vi "TableReceiverGoToSkill.vi"(7 "Firstcall?":bool=TRUE, 8 "error in (no error)":errorcluster, 9 "Game":refnum<class "Game.lvclass">, 10 "Robot in":refnum<class "Robot.lvclass">, 11 "TableReceiverGoToSkill in":refnum<class "TableReceiverGoToSkill.lvclass">) -> (0 "error out":errorcluster, 2 "Robot out":refnum<class "Robot.lvclass">, 3 "TableReceiverGoToSkill out":refnum<class "TableReceiverGoToSkill.lvclass">)   [LabVIEW 2023, in "TableReceiverGoToSkill.lvclass"]
uses:
  TableReceiverGoToSkill.lvclass
  Game_class/Game.lvclass
  Robot_class/Robot.lvclass
  Robot_class/roles.ctl
  Game_class/Game.lvclass/Game.ctl
  Object_class/Object.lvclass/Object.ctl
  Parameters_class/Parameters.lvclass/Parameters.ctl
  Team_class/Team.lvclass/Team.ctl
  Robot_class/Robot.lvclass/Robot.ctl
  Object_class/Read x.vi
  Object_class/Read y.vi
  Game_class/Read Utilities.lvclass.vi
  Game_class/Read BallRef.vi
  Game_class/Read FieldRef.vi
  Game_class/Read Parameters.lvclass.vi
  Game_class/Read OffensiveTeam.vi
  Team_class/Read OffensivePlay.vi
  Team_class/Read RobotRef.vi
  Parameters_class/Read AttakingOurselves.vi
  Robot_class/Write dest_x.vi
  Robot_class/Write dest_y.vi
  Robot_class/Write dest_orientation.vi
  Ally_class/Ally.lvclass
  Ball_class/Ball.lvclass
  Utilities_class/Utilities.lvclass
  Field_class/Field.lvclass
  Parameters_class/Parameters.lvclass
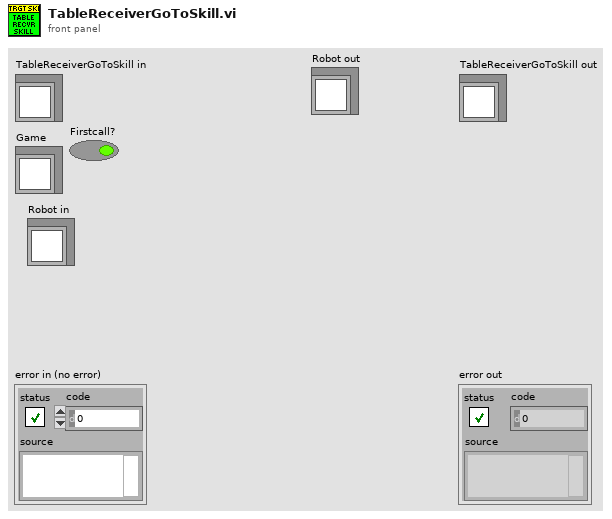
[diagram p1: front panel]
types:
  T1 = typedef "roles.ctl" = enum16{"BallChallengerAttackerVSS", "NormalAttackerVSS", "AttackerAimGoalVSS", "DefenderAreaVSS", "KeeperVSS", "Tabler", "TableFinalizer", "PrepareRollToPassRoller", "PrepareRollToPassReceiver", "SimplePassRoll", "SimplePassRollReceiver", "PenaltyDefense", "PreparePassReceiver 2", "PreparePassReceiver 1", "PassObserver", "Timeout", "Goto", "ZigZag", "None", "BallOutOfField", "DefenderArea", "Duelist", "AttackerStop", "FollowAttacker", "KeeperRole", "KickPenalty", "AttackerAimGoal", "AttackerBlock", "Marker", "Halt", "Shoot", "PassKicker", "PassReceiver", "TestRole", "PenaltyAttacker"}
  T2 = typedef "OffensivePlay.ctl" = enum16{"TableWithStriker", "TableWith2ndStrikerPlay", "PrepareDoublePass", "PrepareRollToPass", "SimplePass", "PreparePass", "PassToStriker", "BallOutOfField", "PassTo2ndStriker", "StopOffensive", "Prepare Penalty Enemy", "EnemyPossessionAtEnemyField", "EnemyPossesionAtOurField", "TestPlay", "PreparePenaltyAlly", "KickPenaltyAlly", "PrepareKickoffAlly", "PrepareKickoffEnemy", "IndirectEnemy", "DirectEnemy", "NormalGame", "DirectKick", "Pass", "Halt", "Timeout", "PassPlay", "PenaltyEnemy"}
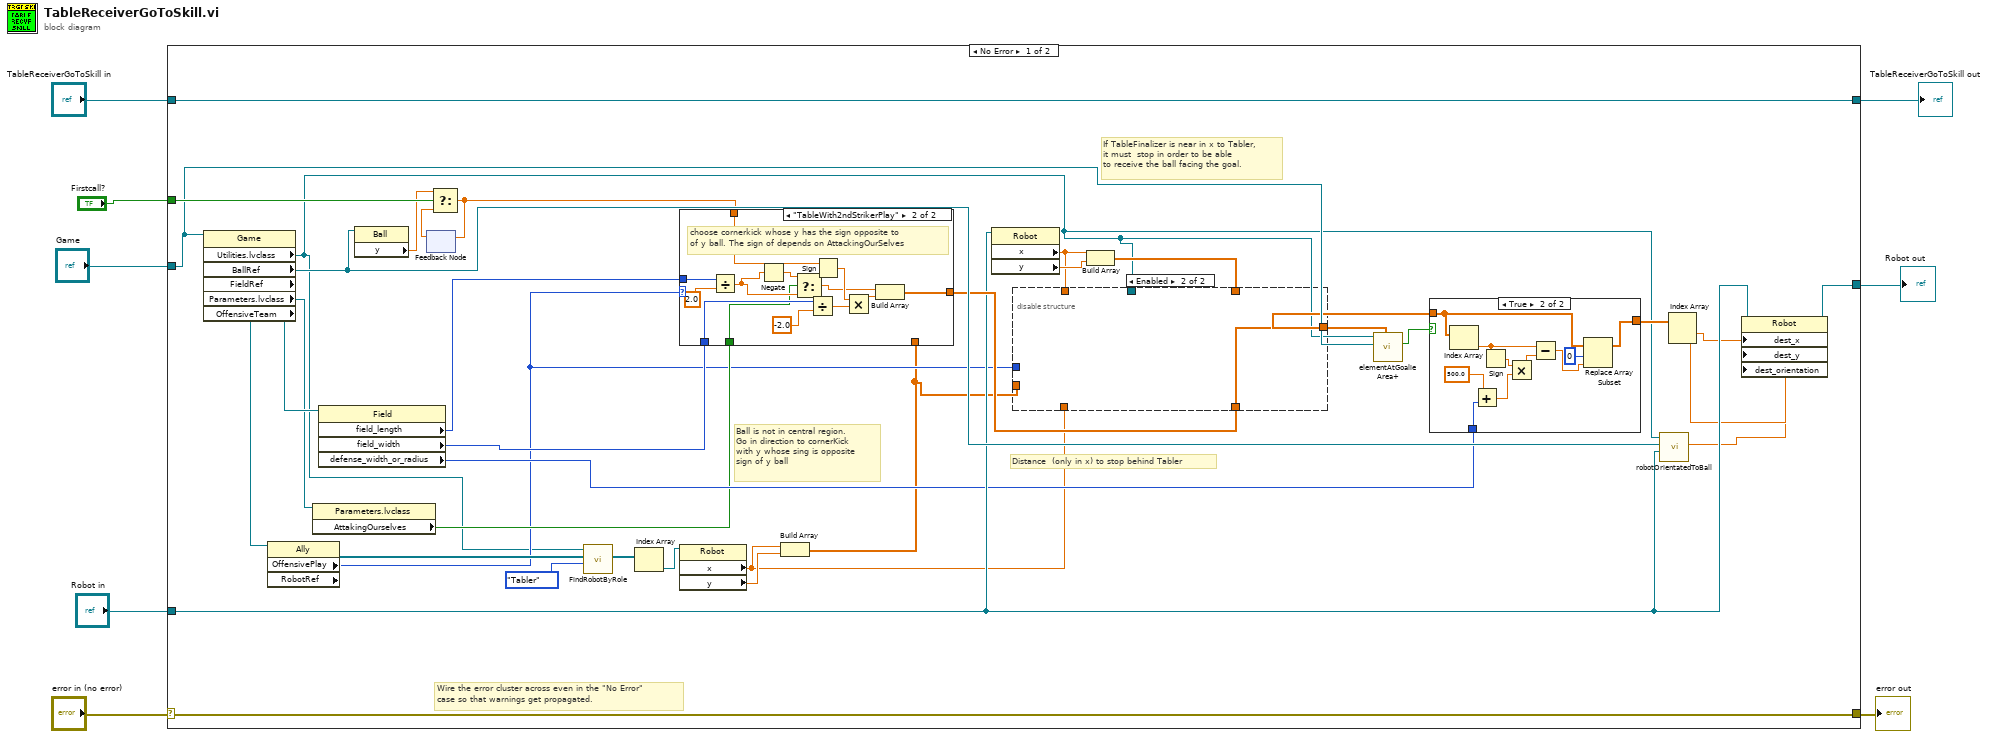
[diagram p0: block diagram]
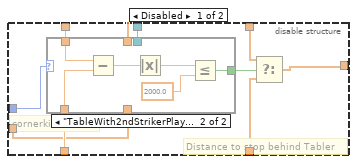
[diagram p2: hidden frame]
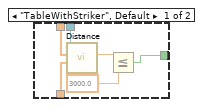
[diagram p3: hidden frame]
diagram:
  n1 = case shown="No Error" "error in (no error)" {
    selector: "error in (no error)" -> [w43 w93]
    tunnel: [w43 w93] -> w7
    tunnel: [w44 w92] -> w5
    tunnel: "TableReceiverGoToSkill in" -> [w44 w92]
    tunnel: "Game" -> [w21 _]
    tunnel: "Robot in" -> [w31 _]
    tunnel: [w27 _] -> w2
    tunnel: "Firstcall?" -> [w26 _]
    frame No Error {
      # "Ball is not in central region.\nGo in direction to cornerKick\nwith y whose sing is opposite\nsign of y ball"
      # "Distance  (only in x) to stop behind Tabler"
      # "If TableFinalizer is near in x to Tabler,\nit must  stop in order to be able\nto receive the ball facing the goal."
      # "Wire the error cluster across even in the \"No Error\"\ncase so that warnings get propagated."
      n2 = property class="Game"(reference=w21) -> ("Utilities.lvclass"=w9:refnum<class "Utilities.lvclass">, "BallRef"=w39:refnum<class "Ball.lvclass">, "FieldRef"=w42:refnum<class "Field.lvclass">, "Parameters.lvclass"=w41:refnum<class "Parameters.lvclass">, "OffensiveTeam"=w33:refnum<class "Ally.lvclass">)  [unwired: 1 in, 2 out]
      n3 = property class="Ally"(reference=w33) -> ("OffensivePlay"=w12:T2, "RobotRef"=w32:refnum<class "Robot.lvclass">[])  [unwired: 1 in, 2 out]
      n4 = property class="Parameters.lvclass"(reference=w41) -> ("AttakingOurselves"=w16:bool)  [unwired: 1 in, 2 out]
      n5 = property class="Field"(reference=w42) -> ("field_length"=w15:i32, "field_width"=w40:i32, "defense_width_or_radius"=w18:i32)  [unwired: 1 in, 2 out]
      n6 = property class="Ball"(reference=w39) -> ("y"=w25:dbl)  [unwired: 1 in, 2 out]
      n7 = feedback #1() -> (w24:dbl)  [unwired: 1 in]
      n8 = Select(t=w25, s=w26, f=w24) -> (s? t:f=w23:dbl)
      n9 = feedback-in #1(w23) -> ()
      n10 = call "FindRobotByRole.vi"("role"=roles."Tabler", "RobotRef"=w32, "Utilities in"=w9) -> ("Robots"=w38:refnum<class "Robot.lvclass">[])  [unwired: 6 in, 2 out]
      n11 = Index Array(array=w38) -> (element=w37:refnum<class "Robot.lvclass">)  [unwired: 1 in]
      n12 = property class="Robot"(reference=w37) -> ("x"=w13:dbl, "y"=w14:dbl)  [unwired: 1 in, 2 out]
      n13 = Build Array(w13, w14) -> (w10:dbl[])
      n14 = case shown="\"TableWith2ndStrikerPlay\"" w12 {
        tunnel: w40 -> [_ w80]
        tunnel: [w67 w79] -> w36
        tunnel: w23 -> [_ w78]
        tunnel: w16 -> [_ w71]
        tunnel: w15 -> [_ w70]
        tunnel: w10 -> [w67 _]
        frame "TableWithStriker", Default {
          # "Go in direction to Tabler"
        }
        frame "TableWith2ndStrikerPlay" {
          # "choose cornerkick whose y has the sign opposite to\nof y ball. The sign of depends on AttackingOurSelves"
          n15 = Divide(x=w70, y=2.0) -> (x/y=w72:dbl)
          n16 = Negate(x=w72) -> (-x=w73:dbl)
          n17 = Select(t=w73, s=w71, f=w72) -> (s? t:f=w69:dbl)
          n18 = Divide(x=w80, y=-2.0) -> (x/y=w75:dbl)
          n19 = Sign(1:w78) -> (0:w76:dbl)
          n20 = Multiply(x=w76, y=w75) -> (x*y=w77:dbl)
          n21 = Build Array(w69, w77) -> (w79:dbl[])
        }
      }
      n22 = property class="Robot"(reference=w31) -> ("x"=w22:dbl, "y"=w35:dbl)  [unwired: 1 in, 2 out]
      n23 = Build Array(w22, w35) -> (w11:dbl[])
      n24 = disable-structure shown="Enabled" {
        disable-tunnel: w36 -> [w52 w66]
        disable-tunnel: w22 -> [w51 _]
        disable-tunnel: [w50 w66] -> w17
        disable-tunnel: w13 -> [w49 _]
        disable-tunnel: w12 -> [w48 _]
        disable-tunnel: w11 -> [w47 _]
        disable-tunnel: w10 -> [w46 _]
        disable-tunnel: w9 -> [w45 _]
        frame Disabled {
          # "Distance to stop behind Tabler"
          # "cornerkick Point"
          n25 = case shown="\"TableWith2ndStrikerPlay\"" w48 {
            tunnel: [w58 w63] -> w53
            tunnel: w51 -> [_ w62]
            tunnel: w49 -> [_ w61]
            tunnel: w47 -> [w56 _]
            tunnel: w46 -> [w57 _]
            tunnel: w45 -> [w55 _]
            frame "TableWithStriker", Default {
              n26 = call-dynamic "Distance.vi"("P1"=w57, "P2"=w56, "Utilities in"=w55) -> ("Distance"=w59:dbl)  [unwired: 6 in, 2 out]
              n27 = Less Or Equal?(x=w59, y=3000.0) -> (x <= y?=w58:bool)
            }
            frame "TableWith2ndStrikerPlay" {
              n28 = Subtract(x=w62, y=w61) -> (x-y=w65:dbl)
              n29 = Absolute Value(x=w65) -> (abs(x)=w64:dbl)
              n30 = Less Or Equal?(x=w64, y=2000.0) -> (x <= y?=w63:bool)
            }
          }
          n31 = Select(t=w47, s=w53, f=w52) -> (s? t:f=w50:dbl[])
        }
        frame Enabled {
        }
      }
      n32 = call "elementAtGoalieArea+.vi"("Elemento pos."=w17, "Game"=w21, "Utilities in"=w9) -> ("Elemento at goalkeeper area + ?"=w20:bool)  [unwired: 6 in, 2 out]
      n33 = case shown="True" w20 {
        tunnel: w17 -> [w81 w90]
        tunnel: [w81 w88] -> w19
        tunnel: w18 -> [_ w82]
        frame False {
        }
        frame True {
          n34 = Index Array(array=w90) -> (element=w87:dbl)  [unwired: 1 in]
          n35 = Add(x=500.0, y=w82) -> (x+y=w84:dbl)
          n36 = Sign(1:w87) -> (0:w89:dbl)
          n37 = Multiply(x=w89, y=w84) -> (x*y=w86:dbl)
          n38 = Subtract(x=w87, y=w86) -> (x-y=w85:dbl)
          n39 = Replace Array Subset(array=w90, new element=w85, index=0) -> (w88:dbl[])
        }
      }
      n40 = call "robotOrientatedToBall.vi"("Robot"=w31, "BallRef"=w39, "Utilities in"=w9) -> ("Orientation"=w28:dbl)  [unwired: 6 in, 2 out]
      n41 = Index Array(array=w19) -> (element #1=w30:dbl, element #2=w29:dbl)  [unwired: 2 in]
      n42 = property class="Robot"(reference=w31, "dest_x"=w30, "dest_y"=w29, "dest_orientation"=w28) -> (reference out=w27:refnum<class "Robot.lvclass">)  [unwired: 1 in, 1 out]
    }
    frame Error {
    }
  }
  "error out" <- w7
  "TableReceiverGoToSkill out" <- w5
  "Robot out" <- w2
